vi "Configure Balance Unbalance Conversion.vi"(0 "VISA resource name":refnum<visa-resource-name>, 1 "Channel (1)":i32=1, 2 "Trace (1)":i32=1, 5 "Conversion State (F: Disable)":bool, 7 "Parameter (0:SSS)":u16(ring) items=["SSS", "SDS", "SSD", "SCS", "SSC", "SDD", "SCD", "SDC", "SCC", "Imbalance 1", "Imbalance 2", "Imbalance 3", "Imbalance 4", "CMRR1", "CMRR2"], 9 "Balance Device Type (0: Unbalance - Balance)":u16(ring) items=["Unbalance - Balance", "Balance - Balance", "Unbalance - Unbalance - Balance"], 11 "error in (no error)":errorcluster, 12 "Port 1 (1)":i32=1, 13 "Port 2 (1)":i32=1) -> (4 "VISA resource name out":refnum<visa-resource-name>, 15 "error out":errorcluster)   [LabVIEW 2020, in "Agilent ENA Series.lvlib"]
doc: "Configures the balance unbalance conversion.\n\n<b>Note:</b>\nFor 5063A, E5072A, E5080A and E5080B unbalance settings are not used."
uses:
  <instrlib>/Agilent ENA Series/Agilent ENA Series.lvlib
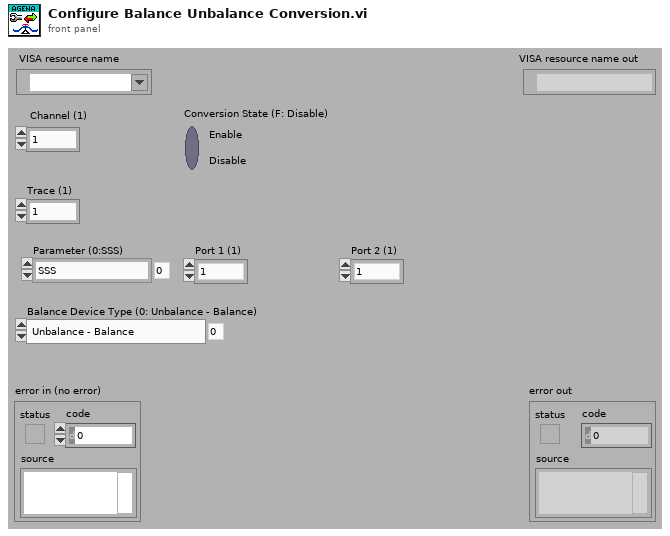
[diagram p1: front panel]
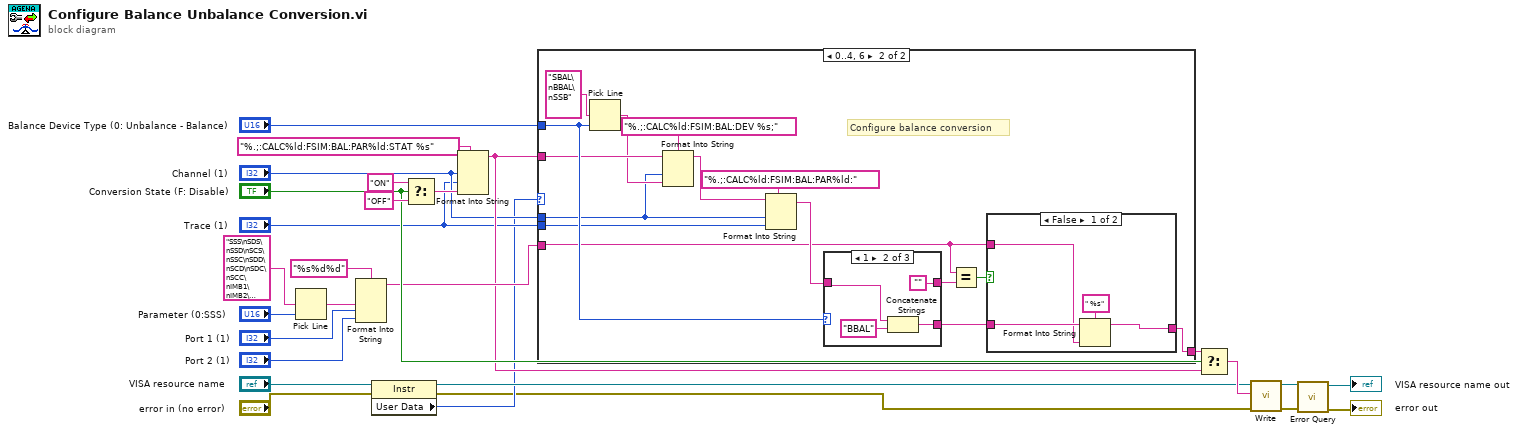
[diagram p0: block diagram]
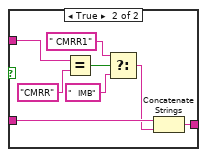
[diagram p3: hidden frame]
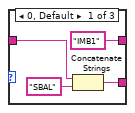
[diagram p4: hidden frame]
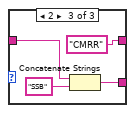
[diagram p5: hidden frame]
diagram:
  n1 = Pick Line(multi-line string="SSS\nSDS\nSSD\nSCS\nSSC\nSDD\nSCD\nSDC\nSCC\nIMB1\nIMB2\nIMB3\nIMB4\nCMRR\nCMRR2", line index="Parameter (0:SSS)") -> (output string=w15:string)  [unwired: 1 in]
  n2 = Format Into String(format string="%s%d%d", w15, "Port 1 (1)", "Port 2 (1)") -> (resulting string=w12:string)  [unwired: 2 in, 1 out]
  n3 = property class="Instr"(reference="VISA resource name", error in="error in (no error)") -> (reference out=w7:refnum<visa-resource-name>, error out=w1:errorcluster, "User Data"=w3:u32)
  n4 = Select(t="ON", s="Conversion State (F: Disable)", f="OFF") -> (s? t:f=w22:string)
  n5 = Format Into String(format string="%.;:CALC%ld:FSIM:BAL:PAR%ld:STAT %s", "Channel (1)", "Trace (1)", w22) -> (resulting string=w6:string)  [unwired: 2 in, 1 out]
  n6 = case shown="0..4, 6" w3 {
    tunnel: "Balance Device Type (0: Unbalance - Balance)" -> [_ w41]
    tunnel: [w28 w36] -> w21
    tunnel: w12 -> [_ w35]
    tunnel: w6 -> [w28 w33]
    tunnel: "Channel (1)" -> [_ w30]
    tunnel: "Trace (1)" -> [_ w29]
    frame 5, 7, Default {
      # "If ENA 5072A or 5063A, none of the unbalance settings are used."
    }
    frame 0..4, 6 {
      # "Configure balance conversion"
      n7 = Pick Line(multi-line string="SBAL\nBBAL\nSSB", line index=w41) -> (output string=w31:string)  [unwired: 1 in]
      n8 = Format Into String(format string="%.;:CALC%ld:FSIM:BAL:DEV %s;", initial string=w33, w30, w31) -> (resulting string=w32:string)  [unwired: 1 in, 1 out]
      n9 = Format Into String(format string="%.;:CALC%ld:FSIM:BAL:PAR%ld:", initial string=w32, w30, w29) -> (resulting string=w40:string)  [unwired: 1 in, 1 out]
      n10 = case shown="1" w41 {
        tunnel: w40 -> [w59 w61 w66]
        tunnel: [w57 w63 w67] -> w37
        tunnel: ["IMB1" "" "CMRR"] -> w39
        frame 0, Default {
          n11 = Concatenate Strings(w59, "SBAL" ("format string")) -> (w57:string)
        }
        frame 1 {
          n12 = Concatenate Strings(w61, "BBAL" ("format string")) -> (w63:string)
        }
        frame 2 {
          n13 = Concatenate Strings(w66, "SSB" ("format string")) -> (w67:string)
        }
      }
      n14 = Equal?(x=w35, y=w39) -> (x = y?=w38:bool)
      n15 = case shown="False" w38 {
        tunnel: w35 -> [w45 w54]
        tunnel: w37 -> [w47 w50]
        tunnel: [w44 w48] -> w36
        frame False {
          n16 = Format Into String(format string=" %s", initial string=w47, w45) -> (resulting string=w44:string)  [unwired: 1 in, 1 out]
        }
        frame True {
          n17 = Equal?(x=w54, y="CMRR") -> (x = y?=w53:bool)
          n18 = Select(t=" CMRR1", s=w53, f="  IMB") -> (s? t:f=w49:string)
          n19 = Concatenate Strings(w50, w49) -> (w48:string)
        }
      }
    }
  }
  n20 = Select(t=w21, s="Conversion State (F: Disable)", f=w6) -> (s? t:f=w23:string)
  n21 = call <instrlib>:"Write.vi"("error in (no error)"=w1, "String ()"=w23, "VISA resource name"=w7) -> ("error out"=w19:errorcluster, "VISA resource name out"=w20:refnum<visa-resource-name>)  [unwired: 6 in, 1 out]
  n22 = call <instrlib>:"Error Query.vi"("error in (no error)"=w19, "VISA resource name"=w20) -> ("error out"=→"error out":errorcluster, "VISA resource name out"=→"VISA resource name out":refnum<visa-resource-name>)  [unwired: 6 in, 2 out]
